vi "Translator.GatherControls.vi"(8 "error in":errorcluster, 11 "VI ref in":refnum<vi>) -> (0 "error out":errorcluster, 2 "Controls out":T1[](array[typedef]), 3 "VI ref out":refnum<vi>)   [LabVIEW 2019, in "Tools.lvlib"]
uses:
  Tools.lvlib
  Translator.ControlData.ctl
  Translator.ControlTypes.ctl
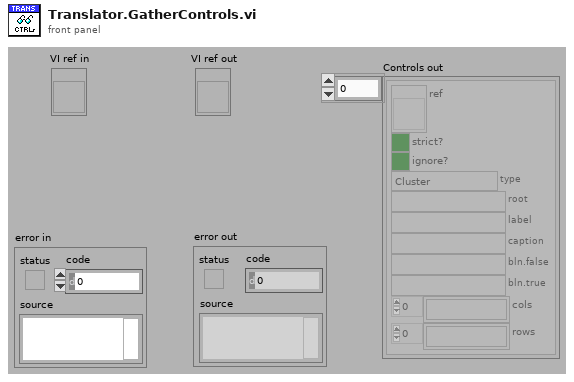
[diagram p1: front panel]
types:
  T1 = typedef "Tools.lvlib/Translator.ControlData.ctl" = cluster{"ref":refnum<vi>, "strict?":bool, "ignore?":bool, "type":T2, "root":string, "label":string, "caption":string, "bln.false":string, "bln.true":string, "cols":string[], "rows":string[]}
  T2 = typedef "Tools.lvlib/Translator.ControlTypes.ctl" = enum16{"Cluster", "Array", "Boolean", "Ring", "String", "Tab", "Listbox", "Multicolumn listbox", "Table", "Other"}
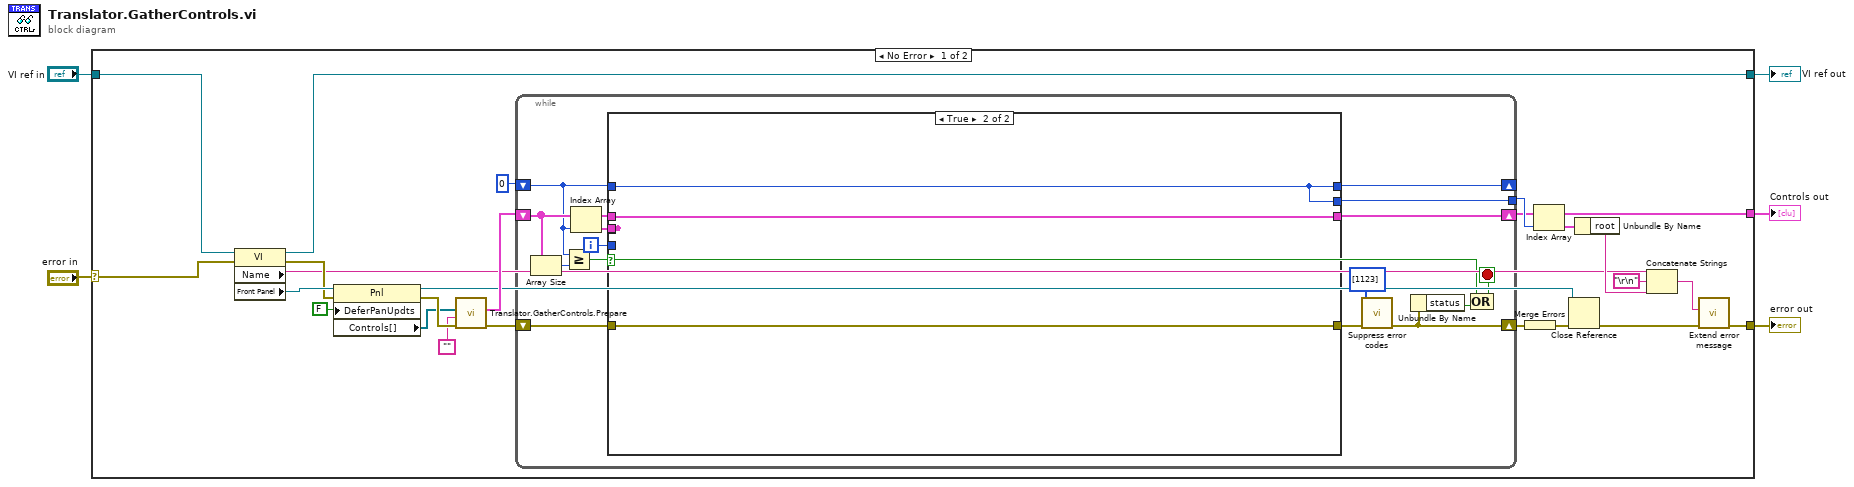
[diagram p0: block diagram]
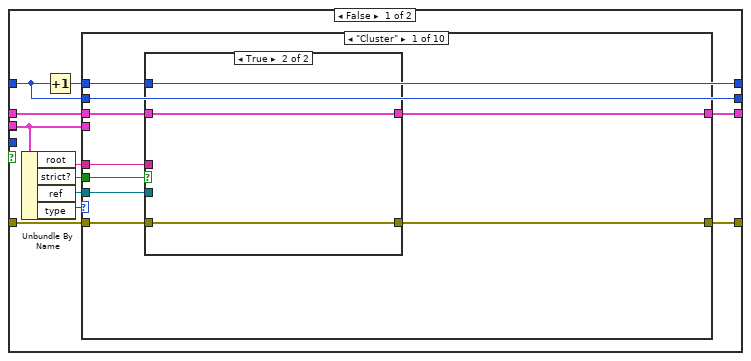
[diagram p2: hidden frame]
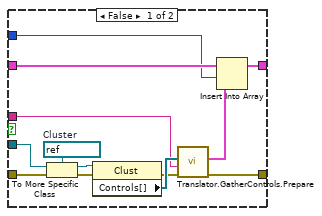
[diagram p3: hidden frame]
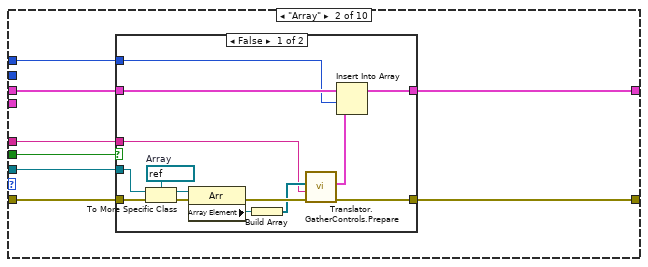
[diagram p4: hidden frame]
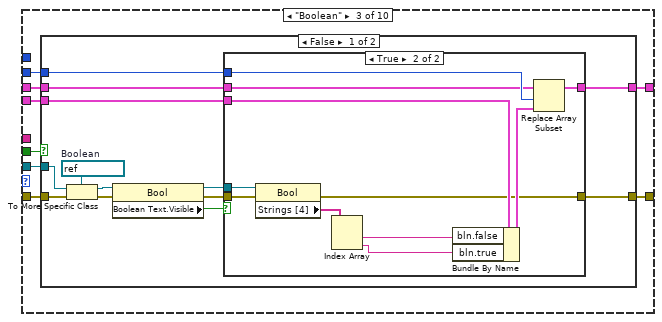
[diagram p6: hidden frame]
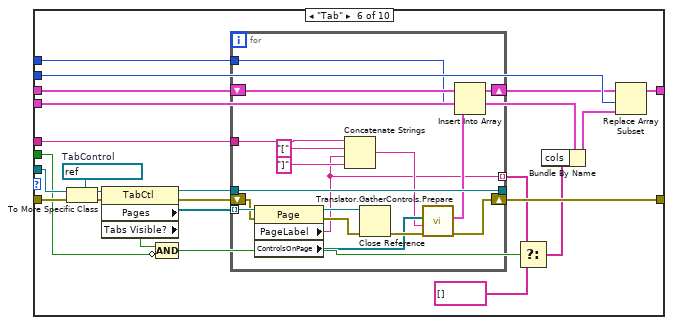
[diagram p11: hidden frame]
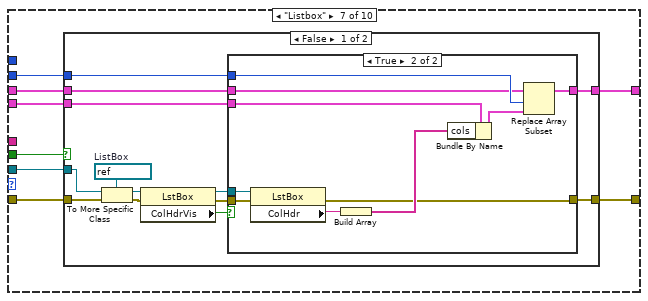
[diagram p12: hidden frame]
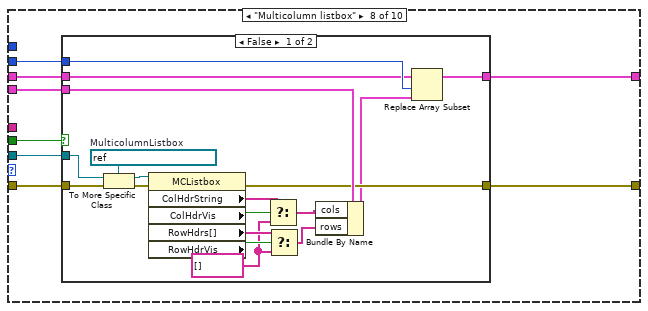
[diagram p15: hidden frame]
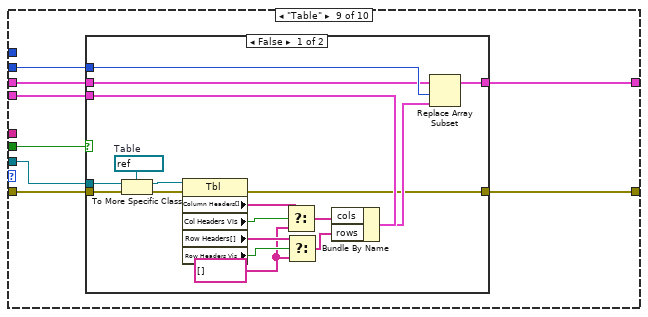
[diagram p17: hidden frame]
diagram:
  n1 = case shown="No Error" "error in" {
    selector: "error in" -> [w10 w280]
    tunnel: [w20 w280] -> w4
    tunnel: [w11 _] -> w3
    tunnel: "VI ref in" -> [w8 w279]
    tunnel: [w7 w279] -> w1
    frame No Error {
      n2 = property class="VI"(reference=w8, error in=w10) -> (reference out=w7:refnum<vi>, error out=w28:errorcluster, "Name"=w6:string, "Front Panel"=w29:refnum<vi>)
      n3 = property class="Pnl"(reference=w29, error in=w28, "DeferPanUpdts"=FALSE ("Defer Panel Updates")) -> (reference out=w21:refnum<vi>, error out=w25:errorcluster, "Controls[]"=w17:refnum<vi>[])
      n4 = call "Translator.GatherControls.Prepare.vi"("error in"=w25, "root"="", "Controls in"=w17) -> ("error out"=w24:errorcluster, "Controls out"=w26:T1[])  [unwired: 7 in]
      n5 = while {
        shift-right: [w40] -> w11
        shift-left: w26 -> [w41]
        shift-right: [w37] -> _
        shift-left: 0 -> [w39]
        tunnel: [w38] -> w18
        shift-right: [w33] -> w22
        shift-left: w24 -> [w42]
        i -> [w30]
        stop <- w34 stop-if-true
        n6 = Array Size(array=w41) -> (size(s)=w44:i32)
        n7 = Greater Or Equal?(x=w39, y=w44) -> (x >= y?=w35:bool)
        n8 = Index Array(array=w41, index=w39) -> (element=w31:T1)
        n9 = case shown="True" w35 {
          tunnel: w31 -> [w46 _]
          tunnel: w42 -> [w53 w277]
          tunnel: w41 -> [w52 w278]
          tunnel: w39 -> [w47 w276]
          tunnel: [w45 w278] -> w40
          tunnel: [w51 w277] -> w36
          tunnel: [w47 w276] -> w38
          tunnel: [w50 w276] -> w37
          tunnel: w31 -> [_ _]
          tunnel: w30 -> [_ _]
          frame False {
            n10 = Unbundle By Name(w46) -> ("root"=w48:string, "strict?"=w49:bool, "ref"=w54:refnum<vi>, "type"=w55:T2)
            n11 = Increment(x=w47) -> (x+1=w50:i32)
            n12 = case shown="\"Cluster\"" w55 {
              tunnel: w54 -> [w63 w86 w109 _ _ w159 w189 w224 w252 _]
              tunnel: w53 -> [w62 w85 w110 w139 w141 w160 w190 w225 w253 w274]
              tunnel: w52 -> [w61 w84 w106 w140 w142 w158 w185 w220 w248 w275]
              tunnel: w50 -> [w60 w83 _ _ _ w157 _ _ _ _]
              tunnel: w49 -> [w56 w79 w103 _ _ w147 w183 w218 w246 _]
              tunnel: w46 -> [_ _ w108 _ _ w156 w188 w223 w251 _]
              tunnel: w47 -> [_ _ w107 _ _ w155 w187 w222 w250 _]
              tunnel: [w59 w82 w105 w140 w142 w152 w186 w221 w249 w275] -> w45
              tunnel: [w58 w81 w104 w139 w141 w151 w184 w219 w247 w274] -> w51
              tunnel: w48 -> [w57 w80 _ _ _ w150 _ _ _ _]
              frame "Cluster" {
                n13 = case shown="True" w56 {
                  tunnel: w63 -> [w75 _]
                  tunnel: [w66 w78] -> w58
                  tunnel: w62 -> [w72 w78]
                  tunnel: w61 -> [w71 w77]
                  tunnel: [w69 w77] -> w59
                  tunnel: w60 -> [w65 _]
                  tunnel: w57 -> [w64 _]
                  frame False {
                    w76 = refnum<vi> refnum  # Cluster
                    n14 = To More Specific Class(target class=w76, reference=w75, error in=w72) -> (specific class reference=w74:refnum<vi>, error out=w73:errorcluster)
                    n15 = property class="Clust"(reference=w74, error in=w73) -> (error out=w67:errorcluster, "Controls[]"=w70:refnum<vi>[])  [unwired: 1 out]
                    n16 = call "Translator.GatherControls.Prepare.vi"("error in"=w67, "root"=w64, "Controls in"=w70) -> ("error out"=w66:errorcluster, "Controls out"=w68:T1[])  [unwired: 7 in]
                    n17 = Insert Into Array(array=w71, index=w65, new element=w68) -> (w69:T1[])
                  }
                  frame True {
                  }
                }
              }
              frame "Array" {
                n18 = case shown="False" w79 {
                  tunnel: w86 -> [w100 _]
                  tunnel: [w91 w102] -> w81
                  tunnel: w85 -> [w97 w102]
                  tunnel: w84 -> [w96 w101]
                  tunnel: [w94 w101] -> w82
                  tunnel: w83 -> [w90 _]
                  tunnel: w80 -> [w87 _]
                  frame False {
                    w89 = refnum<vi> refnum  # Array
                    n19 = To More Specific Class(target class=w89, reference=w100, error in=w97) -> (specific class reference=w99:refnum<vi>, error out=w98:errorcluster)
                    n20 = property class="Arr"(reference=w99, error in=w98) -> (error out=w92:errorcluster, "Array Element"=w95:refnum<vi>)  [unwired: 1 out]
                    n21 = Build Array(w95) -> (w88:refnum<vi>[])
                    n22 = call "Translator.GatherControls.Prepare.vi"("error in"=w92, "root"=w87, "Controls in"=w88) -> ("error out"=w91:errorcluster, "Controls out"=w93:T1[])  [unwired: 7 in]
                    n23 = Insert Into Array(array=w96, index=w90, new element=w93) -> (w94:T1[])
                  }
                  frame True {
                  }
                }
              }
              frame "Boolean" {
                n24 = case shown="False" w103 {
                  tunnel: w110 -> [w120 w137]
                  tunnel: w109 -> [w119 _]
                  tunnel: w108 -> [w118 _]
                  tunnel: w107 -> [w117 _]
                  tunnel: w106 -> [w116 w138]
                  tunnel: [w115 w138] -> w105
                  tunnel: [w111 w137] -> w104
                  frame False {
                    w123 = refnum<vi> refnum  # Boolean
                    n25 = To More Specific Class(target class=w123, reference=w119, error in=w120) -> (specific class reference=w122:refnum<vi>, error out=w121:errorcluster)
                    n26 = property class="Bool"(reference=w122, error in=w121) -> (reference out=w112:refnum<vi>, error out=w113:errorcluster, "Boolean Text.Visible"=w114:bool)
                    n27 = case shown="True" w114 {
                      tunnel: w118 -> [_ w136]
                      tunnel: w117 -> [_ w132]
                      tunnel: w116 -> [w125 w131]
                      tunnel: [w125 w130] -> w115
                      tunnel: w113 -> [w124 w129]
                      tunnel: w112 -> [_ w128]
                      tunnel: [w124 w127] -> w111
                      frame False {
                      }
                      frame True {
                        n28 = property class="Bool"(reference=w128, error in=w129) -> (error out=w127:errorcluster, "Strings [4]"=w126:string[])  [unwired: 1 out]
                        n29 = Index Array(array=w126) -> (element #1=w135:string, element #2=w134:string)  [unwired: 2 in]
                        n30 = Bundle By Name(cluster=w136, "bln.false"=w135, "bln.true"=w134) -> (w133:T1)
                        n31 = Replace Array Subset(array=w131, new element=w133, index=w132) -> (w130:T1[])
                      }
                    }
                  }
                  frame True {
                  }
                }
              }
              frame "String" {
              }
              frame "Ring" {
              }
              frame "Tab" {
                w165 = refnum<vi> refnum  # TabControl
                n32 = To More Specific Class(target class=w165, reference=w159, error in=w160) -> (specific class reference=w161:refnum<vi>, error out=w164:errorcluster)
                n33 = property class="TabCtl"(reference=w161, error in=w164) -> (reference out=w162:refnum<vi>, error out=w163:errorcluster, "Pages"=w143:refnum<vi>[], "Tabs Visible?"=w146:bool)
                n34 = Compound Arithmetic op=AND(w146, invert w147) -> (w145:bool)
                n35 = for {
                  tunnel: w143 -> [w181] mode=indexing
                  tunnel: w162 -> [w182]
                  tunnel: [w182] -> _
                  shift-right: [w171] -> w151
                  shift-left: w163 -> [w180]
                  shift-right: [w173] -> w154
                  shift-left: w158 -> [w175]
                  tunnel: w157 -> [w172]
                  tunnel: [w166] -> w149 mode=indexing
                  tunnel: w150 -> [w170]
                  n36 = property class="Page"(reference=w181, error in=w180) -> (reference out=w178:refnum<vi>, error out=w179:errorcluster, "PageLabel"=w166:string, "ControlsOnPage"=w176:refnum<vi>[])
                  n37 = Concatenate Strings(w170, "[" ("string"), w166, "]" ("string")) -> (w167:string)
                  n38 = Close Reference(reference=w178, error in (no error)=w179) -> (error out=w177:errorcluster)
                  n39 = call "Translator.GatherControls.Prepare.vi"("error in"=w177, "root"=w167, "Controls in"=w176) -> ("error out"=w171:errorcluster, "Controls out"=w174:T1[])  [unwired: 7 in]
                  n40 = Insert Into Array(array=w175, index=w172, new element=w174) -> (w173:T1[])
                }
                n41 = Select(t=w149, s=w145, f=string[] [] ("pages/legend")) -> (s? t:f=w148:string[])
                n42 = Bundle By Name(cluster=w156, "cols"=w148) -> (w153:T1)
                n43 = Replace Array Subset(array=w154, new element=w153, index=w155) -> (w152:T1[])
              }
              frame "Listbox" {
                n44 = case shown="False" w183 {
                  tunnel: w190 -> [w200 w217]
                  tunnel: w189 -> [w199 _]
                  tunnel: w188 -> [w198 _]
                  tunnel: w187 -> [w197 _]
                  tunnel: [w196 w216] -> w186
                  tunnel: w185 -> [w195 w216]
                  tunnel: [w192 w217] -> w184
                  frame False {
                    w203 = refnum<vi> refnum  # ListBox
                    n45 = To More Specific Class(target class=w203, reference=w199, error in=w200) -> (specific class reference=w201:refnum<vi>, error out=w202:errorcluster)
                    n46 = property class="LstBox"(reference=w201, error in=w202) -> (reference out=w193:refnum<vi>, error out=w191:errorcluster, "ColHdrVis"=w194:bool)
                    n47 = case shown="True" w194 {
                      tunnel: w198 -> [_ w212]
                      tunnel: w197 -> [_ w215]
                      tunnel: [w204 w214] -> w196
                      tunnel: w195 -> [w204 w213]
                      tunnel: w191 -> [w205 w209]
                      tunnel: w193 -> [_ w208]
                      tunnel: [w205 w206] -> w192
                      frame False {
                      }
                      frame True {
                        n48 = property class="LstBox"(reference=w208, error in=w209) -> (error out=w206:errorcluster, "ColHdr"=w210:string)  [unwired: 1 out]
                        n49 = Build Array(w210) -> (w207:string[])
                        n50 = Bundle By Name(cluster=w212, "cols"=w207) -> (w211:T1)
                        n51 = Replace Array Subset(array=w213, new element=w211, index=w215) -> (w214:T1[])
                      }
                    }
                  }
                  frame True {
                  }
                }
              }
              frame "Multicolumn listbox" {
                n52 = case shown="False" w218 {
                  tunnel: w225 -> [w240 w244]
                  tunnel: w224 -> [w239 _]
                  tunnel: w223 -> [w238 _]
                  tunnel: w222 -> [w237 _]
                  tunnel: [w236 w245] -> w221
                  tunnel: w220 -> [w234 w245]
                  tunnel: [w233 w244] -> w219
                  frame False {
                    w229 = string[] [] ("f")
                    w243 = refnum<vi> refnum  # MulticolumnListbox
                    n53 = To More Specific Class(target class=w243, reference=w239, error in=w240) -> (specific class reference=w241:refnum<vi>, error out=w242:errorcluster)
                    n54 = property class="MCListbox"(reference=w241, error in=w242) -> (error out=w233:errorcluster, "ColHdrString"=w232:string[], "ColHdrVis"=w235:bool, "RowHdrs[]"=w230:string[], "RowHdrVis"=w231:bool)  [unwired: 1 out]
                    n55 = Select(t=w232, s=w235, f=w229) -> (s? t:f=w228:string[])
                    n56 = Select(t=w230, s=w231, f=w229) -> (s? t:f=w227:string[])
                    n57 = Bundle By Name(cluster=w238, "cols"=w228, "rows"=w227) -> (w226:T1)
                    n58 = Replace Array Subset(array=w234, new element=w226, index=w237) -> (w236:T1[])
                  }
                  frame True {
                  }
                }
              }
              frame "Table" {
                n59 = case shown="False" w246 {
                  tunnel: w253 -> [w268 w272]
                  tunnel: w252 -> [w267 _]
                  tunnel: w251 -> [w266 _]
                  tunnel: w250 -> [w265 _]
                  tunnel: [w263 w273] -> w249
                  tunnel: w248 -> [w261 w273]
                  tunnel: [w260 w272] -> w247
                  frame False {
                    w256 = string[] [] ("f")
                    w271 = refnum<vi> refnum  # Table
                    n60 = To More Specific Class(target class=w271, reference=w267, error in=w268) -> (specific class reference=w269:refnum<vi>, error out=w270:errorcluster)
                    n61 = property class="Tbl"(reference=w269, error in=w270) -> (error out=w260:errorcluster, "Column Headers[]"=w259:string[], "Col Headers Vis"=w262:bool, "Row Headers[]"=w257:string[], "Row Headers Vis"=w258:bool)  [unwired: 1 out]
                    n62 = Select(t=w259, s=w262, f=w256) -> (s? t:f=w255:string[])
                    n63 = Select(t=w257, s=w258, f=w256) -> (s? t:f=w254:string[])
                    n64 = Bundle By Name(cluster=w266, "cols"=w255, "rows"=w254) -> (w264:T1)
                    n65 = Replace Array Subset(array=w261, new element=w264, index=w265) -> (w263:T1[])
                  }
                  frame True {
                  }
                }
              }
              frame "Other" {
              }
            }
          }
          frame True {
          }
        }
        n66 = call "Suppress error codes.vi"("error in (no error)"=w36, "suppress codes([43])"=i32[] [1123]) -> ("error out"=w33:errorcluster)  [unwired: 8 in, 1 out]
        n67 = Unbundle By Name(w33) -> ("status"=w43:bool)
        n68 = Compound Arithmetic op=OR(w35, w43) -> (w34:bool)
      }
      n69 = Merge Errors(w22) -> (w13:errorcluster)
      n70 = Index Array(array=w11, index=w18) -> (element=w19:T1)
      n71 = Close Reference(reference=w21, error in (no error)=w13) -> (error out=w9:errorcluster)
      n72 = Unbundle By Name(w19) -> ("root"=w12:string)
      n73 = Concatenate Strings(w6, "\r\n", w12) -> (w14:string)
      n74 = call "Extend error message.vi"("error in"=w9, "extra message part"=w14) -> ("error out"=w20:errorcluster)  [unwired: 9 in]
    }
    frame Error {
    }
  }
  "error out" <- w4
  "Controls out" <- w3
  "VI ref out" <- w1
